vi "Get STRANS.vi"(8 "error in":errorcluster, 10 "Element Branch In":refnum<class "Tree.lvclass">, 11 "Referential.lvclass In":refnum<class "Referential.lvclass">) -> (0 "error out":errorcluster, 2 "Element Branch out":refnum<class "Tree.lvclass">, 3 "Referential.lvclass Out":refnum<class "Referential.lvclass">)   [LabVIEW 2019, in "ParseGDSII.lvclass"]
uses:
  ParseGDSII.lvclass
  Tree/Tree.lvclass
  DataTypes/Base/GDSII.DataType.lvclass
  Elements/Referential.lvclass
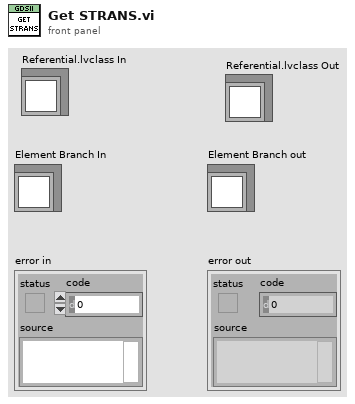
[diagram p1: front panel]
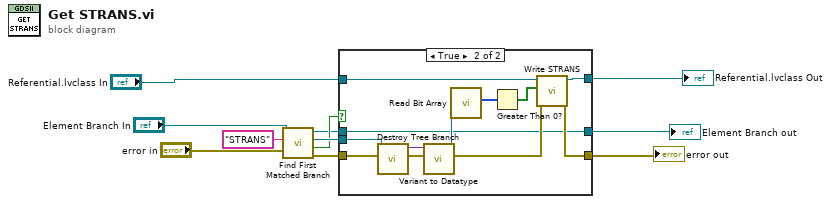
[diagram p0: block diagram]
diagram:
  n1 = call "Find First Matched Branch.vi"("error in"="error in", "Branch Name Exact"="STRANS", "Tree in"="Element Branch In") -> ("error out"=w9:errorcluster, "Found?"=w8:bool, "Matched Branch"=w10:refnum<class "Tree.lvclass">, "Tree out"=w7:refnum<class "Tree.lvclass">)  [unwired: 5 in]
  n2 = case shown="True" w8 {
    tunnel: w10 -> [_ w25]
    tunnel: w9 -> [w13 w23]
    tunnel: [w13 w21] -> w1
    tunnel: "Referential.lvclass In" -> [w14 w20]
    tunnel: [w14 w16] -> w6
    tunnel: [w12 w15] -> w5
    tunnel: w7 -> [w12 w15]
    frame False {
    }
    frame True {
      n3 = call "Destroy Tree Branch.vi"("error in"=w23, "Tree in"=w25) -> ("error out"=w24:errorcluster, "Root"=w26:variant)  [unwired: 8 in]
      n4 = call "Variant to Datatype.vi"("error in"=w24, "Variant"=w26) -> ("error out"=w22:errorcluster, "DataType"=w19:refnum<class "GDSII.DataType.lvclass">)  [unwired: 8 in]
      n5 = call-dynamic "Read Bit Array.vi"("GDSII.DataType in"=w19) -> ("Bit Array"=w18:i16[])  [unwired: 9 in, 1 out]
      n6 = Greater Than 0?(x=w18) -> (x > 0?=w17:bool[])
      n7 = call-dynamic "Write STRANS.vi"("error in (no error)"=w22, "STRANS"=w17, "Referential in"=w20) -> ("error out"=w21:errorcluster, "Referential out"=w16:refnum<class "Referential.lvclass">)  [unwired: 7 in]
    }
  }
  "Element Branch out" <- w5
  "Referential.lvclass Out" <- w6
  "error out" <- w1
